vi "Convolution_kernel.vi"(11 "kernel Enum":T1(ring)) -> (3 "laplacian operator":sgl[][](array[numeric]))   [LabVIEW 2018]
panel:
  # "1、模糊（blur）\n\n模糊内核消除了相邻像素值之间的差异。内核如下：\n\n0.0625\t0.125\t0.0625\n0.125\t0.25\t0.125\n0.0625\t0.125\t0.125"
  # "2、索贝尔（sobel）\nsobel内核用于仅显示特定方向上相邻像素值的差异，分为left sobel、right sobel（检测梯度的水平变化）、top sobel、buttom sobel（检测梯度的垂直变化）。\n例如，buttom sobel\n-1\t-2\t-1\n0\t0\t0\n1\t2\t1"
  # "3、浮雕（emboss）\n\n通过强调像素的差在给定方向的Givens深度的错觉。在这种情况下，沿着从左上到右下的直线的方向。\n\n-2\t-1\t0\n-1\t1\t1\n0\t1\t2"
  # "4、大纲（outline）\n一个轮廓内核（也称为“边缘”的内核）用于突出显示的像素值大的差异。具有接近相同强度的相邻像素旁边的像素在新图像中将显示为黑色，而与强烈不同的相邻像素相邻的像素将显示为白色。\n-1\t-1\t-1\n-1\t8\t-1\n-1\t-1\t-1"
  # "5、锐化（sharpen）\n\n该锐化内核强调在相邻的像素值的差异。这使图像看起来更生动。\n\n0\t-1\t0\n-1\t5\t-1\n0\t-1\t0"
  # "6、拉普拉斯算子（laplacian operator）\n拉普拉斯算子可以用于边缘检测，对于检测图像中的模糊也非常有用。\n\n0\t1\t0\n1\t-4\t1\n0\t1\t0"
  # "7、分身（identity）\n这个非常简单，就是原图（不考虑边界时），How boring!\n\n0\t0\t0\n0\t1\t0\n0\t0\t0"
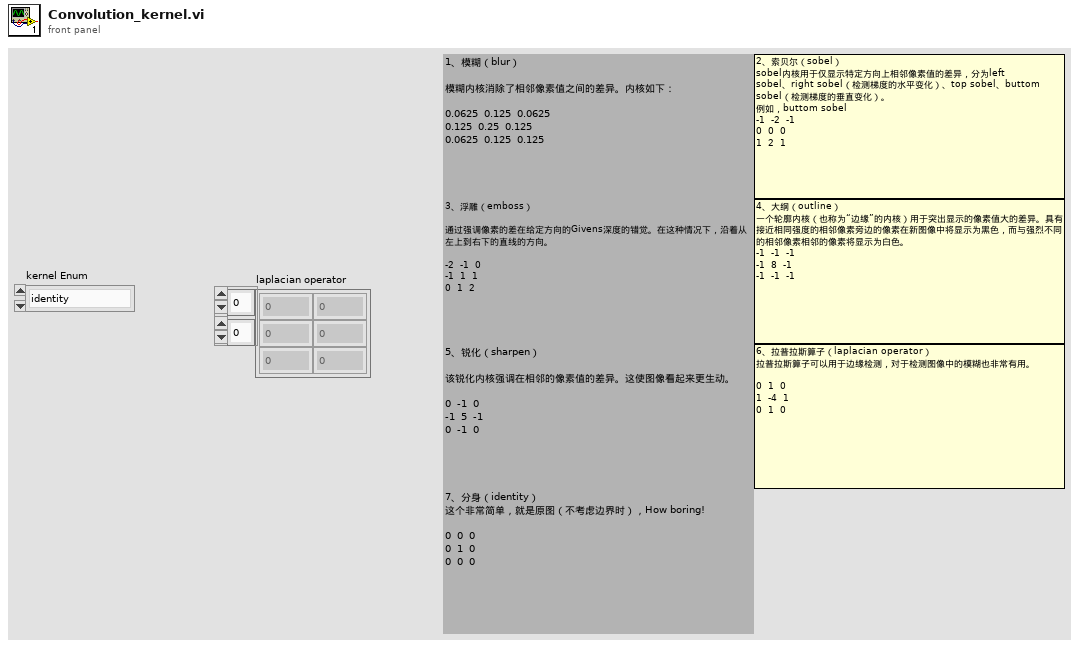
[diagram p1: front panel]
types:
  T1 = enum16{"identity", "outline", "blur", "sobel", "emboss", "sharpen", "laplacian operator"}
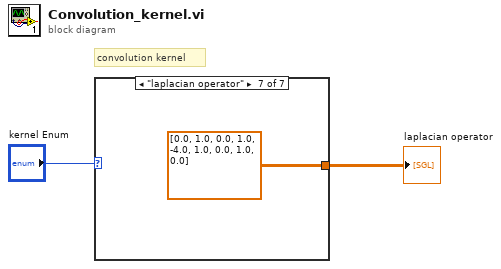
[diagram p0: block diagram]
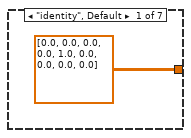
[diagram p2: hidden frame]
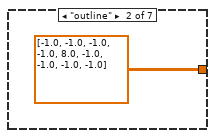
[diagram p3: hidden frame]
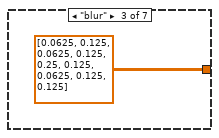
[diagram p4: hidden frame]
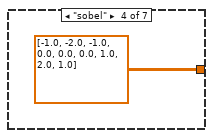
[diagram p5: hidden frame]
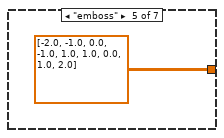
[diagram p6: hidden frame]
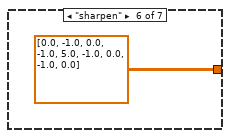
[diagram p7: hidden frame]
diagram:
  # "convolution kernel"
  n1 = case shown="\"laplacian operator\"" "kernel Enum" {
    tunnel: [sgl[][] [[0.0, 0.0, 0.0], [0.0, 1.0, 0.0], [0.0, 0.0, 0.0]] ("identity") sgl[][] [[-1.0, -1.0, -1.0], [-1.0, 8.0, -1.0], [-1.0, -1.0, -1.0]] ("outline") sgl[][] [[0.0625, 0.125, 0.0625], [0.125, 0.25, 0.125], [0.0625, 0.125, 0.125]] ("blur") sgl[][] [[-1.0, -2.0, -1.0], [0.0, 0.0, 0.0], [1.0, 2.0, 1.0]] ("sobel") sgl[][] [[-2.0, -1.0, 0.0], [-1.0, 1.0, 1.0], [0.0, 1.0, 2.0]] ("emboss") sgl[][] [[0.0, -1.0, 0.0], [-1.0, 5.0, -1.0], [0.0, -1.0, 0.0]] ("sharpen") sgl[][] [[0.0, 1.0, 0.0], [1.0, -4.0, 1.0], [0.0, 1.0, 0.0]] ("laplacian operator")] -> w1
    frame "identity", Default {
    }
    frame "outline" {
    }
    frame "blur" {
    }
    frame "sobel" {
    }
    frame "emboss" {
    }
    frame "sharpen" {
    }
    frame "laplacian operator" {
    }
  }
  "laplacian operator" <- w1
